vi "Get Call Chain.vi"(8 "error in (no error)":errorcluster, 11 "Record.Error in":refnum<class "Record.Error.lvclass">) -> (0 "error out":errorcluster, 2 "Call Chain":string, 3 "Record.Error out":refnum<class "Record.Error.lvclass">)   [LabVIEW 2017, in "Error Log.lvlib" / "Record.Error.lvclass"]
uses:
  Record.Error.lvclass
  Record.Error.lvclass/Record.Error.ctl
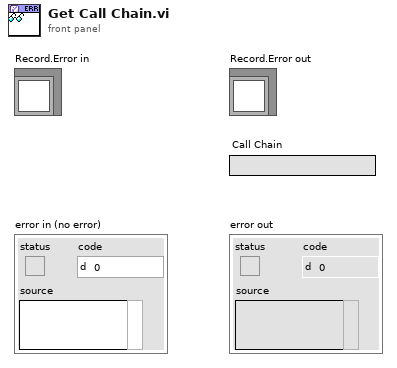
[diagram p1: front panel]
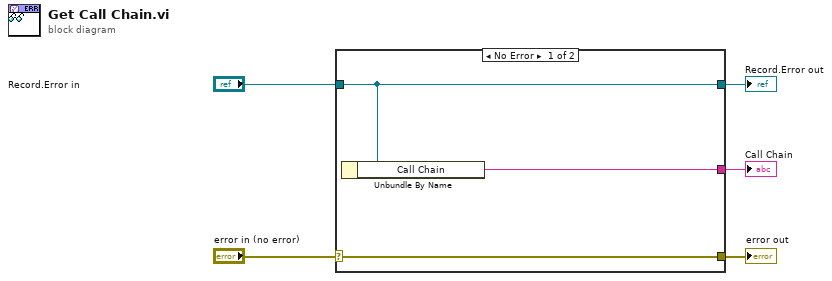
[diagram p0: block diagram]
diagram:
  n1 = case shown="No Error" "error in (no error)" {
    selector: "error in (no error)" -> [w8 w9]
    tunnel: [w8 w9] -> w4
    tunnel: [w7 w10] -> w2
    tunnel: "Record.Error in" -> [w7 w10]
    tunnel: [w6 _] -> w1
    frame No Error {
      n2 = Unbundle By Name(w7) -> ("Call Chain"=w6:string)
    }
    frame Error {
    }
  }
  "error out" <- w4
  "Record.Error out" <- w2
  "Call Chain" <- w1
